vi "DoAction.vi"(8 "error in (no error)":errorcluster, 11 "SimpleDevice in":refnum<class "SimpleDevice.lvclass">) -> (0 "error out":errorcluster, 3 "SimpleDevice out":refnum<class "SimpleDevice.lvclass">)   [LabVIEW 2021, in "SimpleDevice.lvlib" / "SimpleDevice.lvclass"]
uses:
  SimpleDevice.lvclass
  SimpleDevice.lvclass/SimpleDevice.ctl
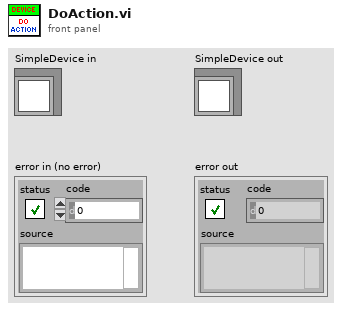
[diagram p1: front panel]
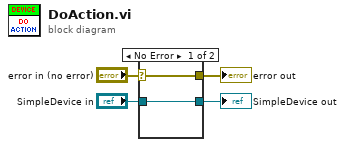
[diagram p0: block diagram]
diagram:
  n1 = case shown="No Error" "error in (no error)" {
    selector: "error in (no error)" -> [w5 w8]
    tunnel: [w5 w8] -> w3
    tunnel: [w6 w7] -> w1
    tunnel: "SimpleDevice in" -> [w6 w7]
    frame No Error {
    }
    frame Error {
    }
  }
  "error out" <- w3
  "SimpleDevice out" <- w1
